vi "set_quantity.vi"(7 "Quantity Name":string, 8 "error in":errorcluster, 11 "Quantity Value":T1) -> (0 "error out":errorcluster)   [LabVIEW 2013]
uses:
  TD Quantity.ctl
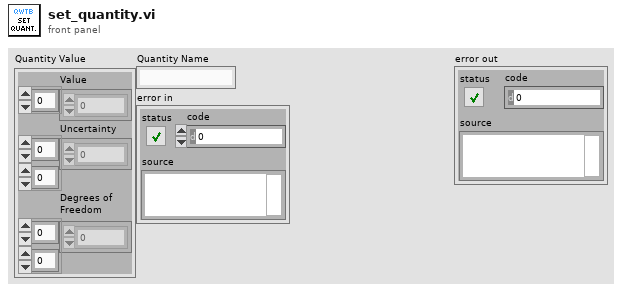
[diagram p1: front panel]
types:
  T1 = typedef "TD Quantity.ctl" = cluster{"Value":dbl[], "Uncertainty":dbl[][], "Degrees of\nFreedom":dbl[][]}
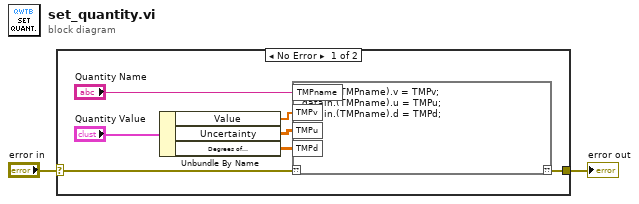
[diagram p0: block diagram]
diagram:
  n1 = case shown="No Error" "error in" {
    selector: "error in" -> [w5 w10]
    tunnel: [w6 w10] -> w2
    frame No Error {
      n2 = Unbundle By Name("Quantity Value") -> ("Value"=w9:dbl[], "Uncertainty"=w8:dbl[][], "Degrees of\nFreedom"=w7:dbl[][])
      n3 = script code="datain.(TMPname).v = TMPv;\ndatain.(TMPname).u = TMPu;\ndatain.(TMPname).d = TMPd;"("??"=w5, "TMPv"=w9, "TMPu"=w8, "TMPd"=w7, "TMPname"="Quantity Name") -> ("??"=w6:errorcluster)
    }
    frame Error {
    }
  }
  "error out" <- w2
